vi "conversionendecimal.vi"(11 "Array":i16[](array[numeric])) -> (0 "resultat en decimal":i16)   [LabVIEW 2019]
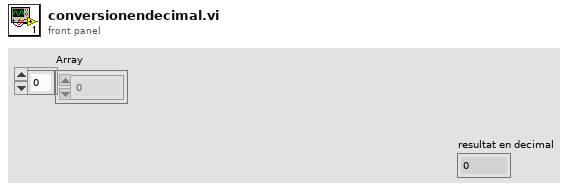
[diagram p1: front panel]
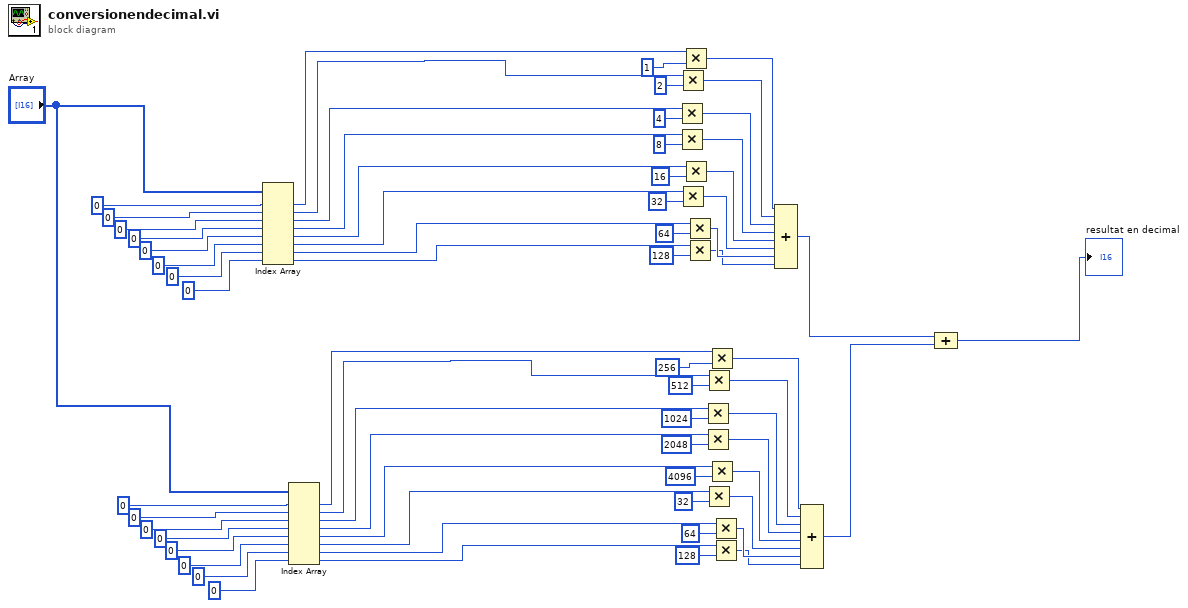
[diagram p0: block diagram]
diagram:
  n1 = Index Array(array="Array", index #1=0 ("index"), index #2=0 ("index"), index #3=0 ("index"), index #4=0 ("index"), index #5=0 ("index"), index #6=0 ("index"), index #7=0 ("index"), index #8=0 ("index")) -> (element #1=w58:i16, element #2=w57:i16, element #3=w54:i16, element #4=w52:i16, element #5=w51:i16, element #6=w50:i16, element #7=w49:i16, element #8=w48:i16)
  n2 = Index Array(array="Array", index #1=0 ("index"), index #2=0 ("index"), index #3=0 ("index"), index #4=0 ("index"), index #5=0 ("index"), index #6=0 ("index"), index #7=0 ("index"), index #8=0 ("index")) -> (element #1=w26:i16, element #2=w25:i16, element #3=w22:i16, element #4=w20:i16, element #5=w19:i16, element #6=w18:i16, element #7=w17:i16, element #8=w16:i16)
  n3 = Multiply(x=w54, y=i16 4) -> (x*y=w42:i16)
  n4 = Multiply(x=w52, y=i16 8) -> (x*y=w41:i16)
  n5 = Multiply(x=w57, y=i16 2) -> (x*y=w55:i16)
  n6 = Multiply(x=w50, y=i16 32) -> (x*y=w39:i16)
  n7 = Multiply(x=w58, y=i16 1) -> (x*y=w59:i16)
  n8 = Multiply(x=w51, y=i16 16) -> (x*y=w40:i16)
  n9 = Multiply(x=w49, y=i16 64) -> (x*y=w38:i16)
  n10 = Multiply(x=w48, y=i16 128) -> (x*y=w37:i16)
  n11 = Multiply(x=w22, y=i16 1024) -> (x*y=w10:i16)
  n12 = Multiply(x=w20, y=i16 2048) -> (x*y=w9:i16)
  n13 = Multiply(x=w25, y=i16 512) -> (x*y=w23:i16)
  n14 = Multiply(x=w18, y=i16 32) -> (x*y=w7:i16)
  n15 = Multiply(x=w26, y=i16 256) -> (x*y=w27:i16)
  n16 = Multiply(x=w19, y=i16 4096) -> (x*y=w8:i16)
  n17 = Multiply(x=w17, y=i16 64) -> (x*y=w6:i16)
  n18 = Multiply(x=w16, y=i16 128) -> (x*y=w5:i16)
  n19 = Compound Arithmetic op=ADD(w59, w55, w42, w41, w40, w39, w38, w37) -> (w2:i16)
  n20 = Compound Arithmetic op=ADD(w27, w23, w10, w9, w8, w7, w6, w5) -> (w3:i16)
  n21 = Compound Arithmetic op=ADD(w2, w3) -> (→"resultat en decimal":i16)
